vi "GenerateSinusoidalOutput.vi"(8 "Init":bool, 10 "Amplitude":dbl=1.0, 11 "Period (s)":dbl=10.0) -> (3 "sin(time)":dbl)   [LabVIEW 2019]
doc: "Generates sinusoidal output with amplitude and period as a function of time"
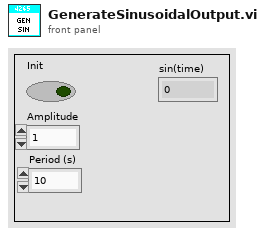
[diagram p1: front panel]
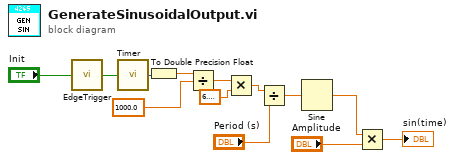
[diagram p0: block diagram]
diagram:
  n1 = call "EdgeTrigger.vi"("Input Signal"="Init") -> ("Rising Edge Trigger"=w11:bool)  [unwired: 2 out]
  n2 = call "Timer.vi"("Reset Timer"=w11) -> ("Time (ms)"=w7:u32)
  n3 = To Double Precision Float(number=w7) -> (double precision float=w8:dbl)
  n4 = Divide(x=w8, y=1000.0) -> (x/y=w5:dbl)
  n5 = Multiply(x=w5, y=6.283185307179586) -> (x*y=w4:dbl)
  n6 = Divide(x=w4, y="Period (s)") -> (x/y=w2:dbl)
  n7 = Sine(x=w2) -> (sin(x)=w13:dbl)
  n8 = Multiply(x=w13, y="Amplitude") -> (x*y=→"sin(time)":dbl)
